vi "distribution_folder_read.vi"(8 "error in (no error)":errorcluster, 11 "lv-builder-default in":refnum<class "lv-builder-default.lvclass">) -> (0 "error out":errorcluster, 2 "distribution_folder":path, 3 "lv-builder-default out":refnum<class "lv-builder-default.lvclass">)   [LabVIEW 2015, in "lv-builder-default.lvclass"]
uses:
  lv-builder-default.lvclass
  lv-builder-default.lvclass/lv-builder-default.ctl
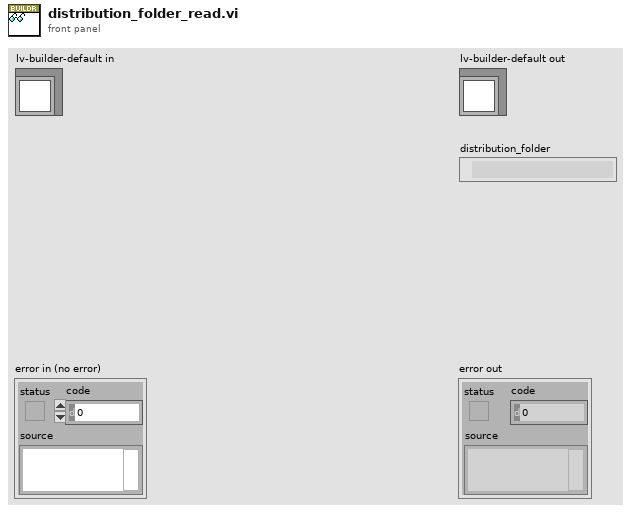
[diagram p1: front panel]
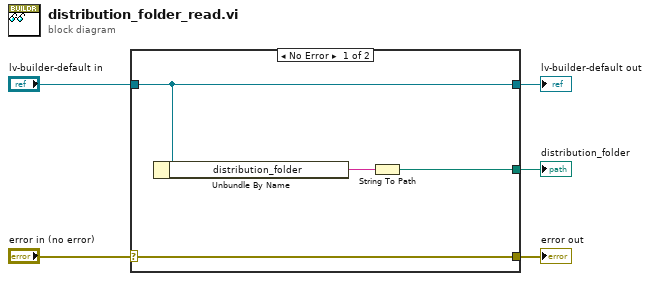
[diagram p0: block diagram]
diagram:
  n1 = case shown="No Error" "error in (no error)" {
    selector: "error in (no error)" -> [w9 w10]
    tunnel: [w9 w10] -> w4
    tunnel: [w8 w11] -> w2
    tunnel: "lv-builder-default in" -> [w8 w11]
    tunnel: [w6 _] -> w1
    frame No Error {
      n2 = Unbundle By Name(w8) -> ("distribution_folder"=w7:string)
      n3 = String To Path(string=w7) -> (path=w6:path)
    }
    frame Error {
    }
  }
  "error out" <- w4
  "lv-builder-default out" <- w2
  "distribution_folder" <- w1
